vi "Plotting Location.vi"(6 "Refresh Rate (ms)":dbl, 7 "Angle":dbl, 8 "Y-Motion":dbl, 9 "Old Y":dbl, 10 "Old X":dbl, 11 "X Motion":dbl) -> (1 "New Y":dbl, 2 "New X":dbl)   [LabVIEW 2015]
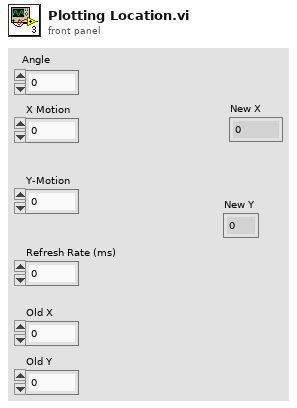
[diagram p1: front panel]
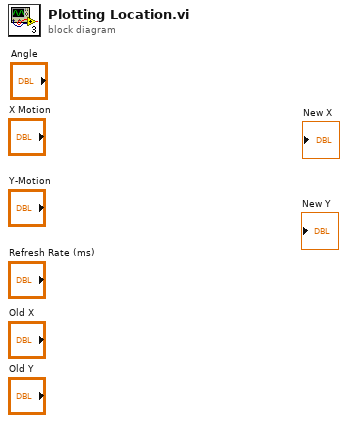
[diagram p0: block diagram]
diagram:
